vi "canDataSortSubVI.vi"(8 "canArrayID_In":string[](array[string]), 9 "canArrayDataIn":string[](array[string]), 11 "dataIn":string="         2  1FFFFFFF   00000004    8        00\t00\tFF\tFF\tFF\tFF\tFF\tFF\r\n         3  0CF101A7   00000004    8        68\t00\t97\tCC\t00\t15\t39\t1A\r\n         2  1FFFFFFF   00000004    8        00\t00\tFF\tFF\tFF\tFF\tFF\tFF\r\n         3  0CF102A7   00000004    8        30\t75\tE0\t2E\t80\tFF\tFF\tFD\r\n         3  0CF101A7   00000004    8        68\t00\t97\tCC\t00\t15\t39\t1A\r\n         2  1FFFFFFF   00000004    8        00\t00\tFF\tFF\tFF\tFF\tFF\tFF\r\n        12  1FFFFFFF   00000004    8        00\t20\tFF\tFF\tFF\tFF\tFF\tFF\r\n         3  0CF102A7   00000004    8        30\t75\tE0\t2E\t80\tFF\tFF\tFD\r\n         3  0CF101A7   00000004    8        68\t00\t97\tCC\t00\t15\t39\t1A\r\n         2  1FFFFFFF   00000004    8        00\t00\tFF\tFF\tFF\tFF\tFF\tFF\r\n        22  1FFFFFFF   00000004    8        00\t20\tFF\tFF\tFF\tFF\tFF\tFF\r\n        12  1FFFFFFF   00000004    8        00\t20\tFF\tFF\tFF\tFF\tFF\tFF\r\n         3  0CF102A7   00000004    8        30\t75\tE0\t2E\t80\tFF\tFF\tFD\r\n         3  0CF101A7   00000004    8        68\t00\t97\tCC\t00\t15\t39\t1A\r\n         2  1FFFFFFF   00000004    8        00\t00\tFF\tFF\tFF\tFF\tFF\tFF\r\n        23  0CF101A7   00000004    8        68\t00\t97\tCC\t00\t15\t39\t1B\r\n        22  1FFFFFFF   00000004    8        00\t20\tFF\tFF\tFF\tFF\tFF\tFF\r\n        12  1FFFFFFF   00000004    8        00\t20\tFF\tFF\tFF\tFF\tFF\tFF\r\n         3  0CF102A7   00000004    8        30\t75\tE0\t2E\t80\tFF\tFF\tFD\r\n         3  0CF101A7   00000004    8        68\t00\t97\tCC\t00\t15\t39\t1A\r\n         2  1FFFFFFF   00000004    8        00\t00\tFF\tFF\tFF\tFF\tFF\tFF\r\n        23  0CF102A7   00000004    8        30\t75\tE0\t2E\t80\tFF\tFF\tFD\r\n        23  0CF101A7   00000004    8        68\t00\t97\tCC\t00\t15\t39\t1B\r\n        22  1FFFFFFF   00000004    8        00\t20\tFF\tFF\tFF\tFF\tFF\tFF\r\n        12  1FFFFFFF   00000004    8        00\t20\tFF\tFF\tFF\tFF\tFF\tFF\r\n         3  0CF102A7   00000004    8        30\t75\tE0\t2E\t80\tFF\tFF\tFD\r\n         3  0CF101A7   00000004    8        68\t00\t97\tCC\t00\t15\t39\t1A\r\n         2  1FFFFFFF   00000004    8        00\t00\tFF\tFF\tFF\tFF\tFF\tFF\r\n        32  1FFFFFFF   00000004    8        00\t20\tFF\tFF\tFF\tFF\tFF\tFF\r\n        23  0CF102A7   00000004    8        30\t75\tE0\t2E\t80\tFF\tFF\tFD\r\n        23  0CF101A7   00000004    8        68\t00\t97\tCC\t00\t15\t39\t1B\r\n        22  1FFFFFFF   00000004    8        00\t20\tFF\tFF\tFF\tFF\tFF\tFF\r\n        12  1FFFFFFF   00000004    8        00\t20\tFF\tFF\tFF\tFF\tFF\tFF\r\n         3  0CF102A7   00000004    8        30\t75\tE0\t2E\t80\tFF\tFF\tFD\r\n         3  0CF101A7   00000004    8        68\t00\t97\tCC\t00\t15\t39\t1A\r\n         2  1FFFFFFF   00000004    8        00\t00\tFF\tFF\tFF\tFF\tFF\tFF\r\n        41  18F11FF0   00000004    8        FF\t3F\t90\t68\t88\t1B\t10\t8C\r\n        32  1FFFFFFF   00000004    8        00\t20\tFF\tFF\tFF\tFF\tFF\tFF\r\n        23  0CF102A7   00000004    8        30\t75\tE0\t2E\t80\tFF\tFF\tFD\r\n        23  0CF101A7   00000004    8        68\t00\t97\tCC\t00\t15\t39\t1B\r\n        22  1FFFFFFF   00000004    8        00\t20\tFF\tFF\tFF\tFF\tFF\tFF\r\n        12  1FFFFFFF   00000004    8        00\t20\tFF\tFF\tFF\tFF\tFF\tFF\r\n         3  0CF102A7   00000004    8        30\t75\tE0\t2E\t80\tFF\tFF\tFD\r\n         3  0CF101A7   00000004    8        68\t00\t97\tCC\t00\t15\t39\t1A\r\n         2  1FFFFFFF   00000004    8        00\t00\tFF\tFF\tFF\tFF\tFF\tFF\r\n        42  18F120F0   00000004    8        2B\t75\t60\tB1\tB0\t01\tFF\tFF\r\n        41  18F11FF0   00000004    8        FF\t3F\t90\t68\t88\t1B\t10\t8C\r\n        32  1FFFFFFF   00000004    8        00\t20\tFF\tFF\tFF\tFF\tFF\tFF\r\n        23  0CF102A7   00000004    8        30\t75\tE0\t2E\t80\tFF\tFF\tFD\r\n        23  0CF101A7   00000004    8        68\t00\t97\tCC\t00\t15\t39\t1B\r\n        22  1FFFFFFF   00000004    8        00\t20\tFF\tFF\tFF\tFF\tFF\tFF\r\n        12  1FFFFFFF   00000004    8        00\t20\tFF\tFF\tFF\tFF\tFF\tFF\r\n         3  0CF102A7   00000004    8        30\t75\tE0\t2E\t80\tFF\tFF\tFD\r\n         3  0CF101A7   00000004    8        68\t00\t97\tCC\t00\t15\t39\t1A\r\n         2  1FFFFFFF   00000004    8        00\t00\tFF\tFF\tFF\tFF\tFF\tFF\r\n        43  0CF101A7   00000004    8        68\t00\t97\tCC\t00\t15\t39\t1C\r\n        42  18F120F0   00000004    8        2B\t75\t60\tB1\tB0\t01\tFF\tFF\r\n        41  18F11FF0   00000004    8        FF\t3F\t90\t68\t88\t1B\t10\t8C\r\n        32  1FFFFFFF   00000004    8        00\t20\tFF\tFF\tFF\tFF\tFF\tFF") -> (1 "canArrayID":string[](array[string]), 3 "canArrayData":string[](array[string]))   [LabVIEW 2023]
panel:
  out "substring":string
  out "arrayIndex":i32
  out "whileIndex":i32
  out "index of element":i32
  out "ID":string[](array[string])
  out "Array 3":string[](array[string])
  # "VCU1:ID=0x0CF101A7"
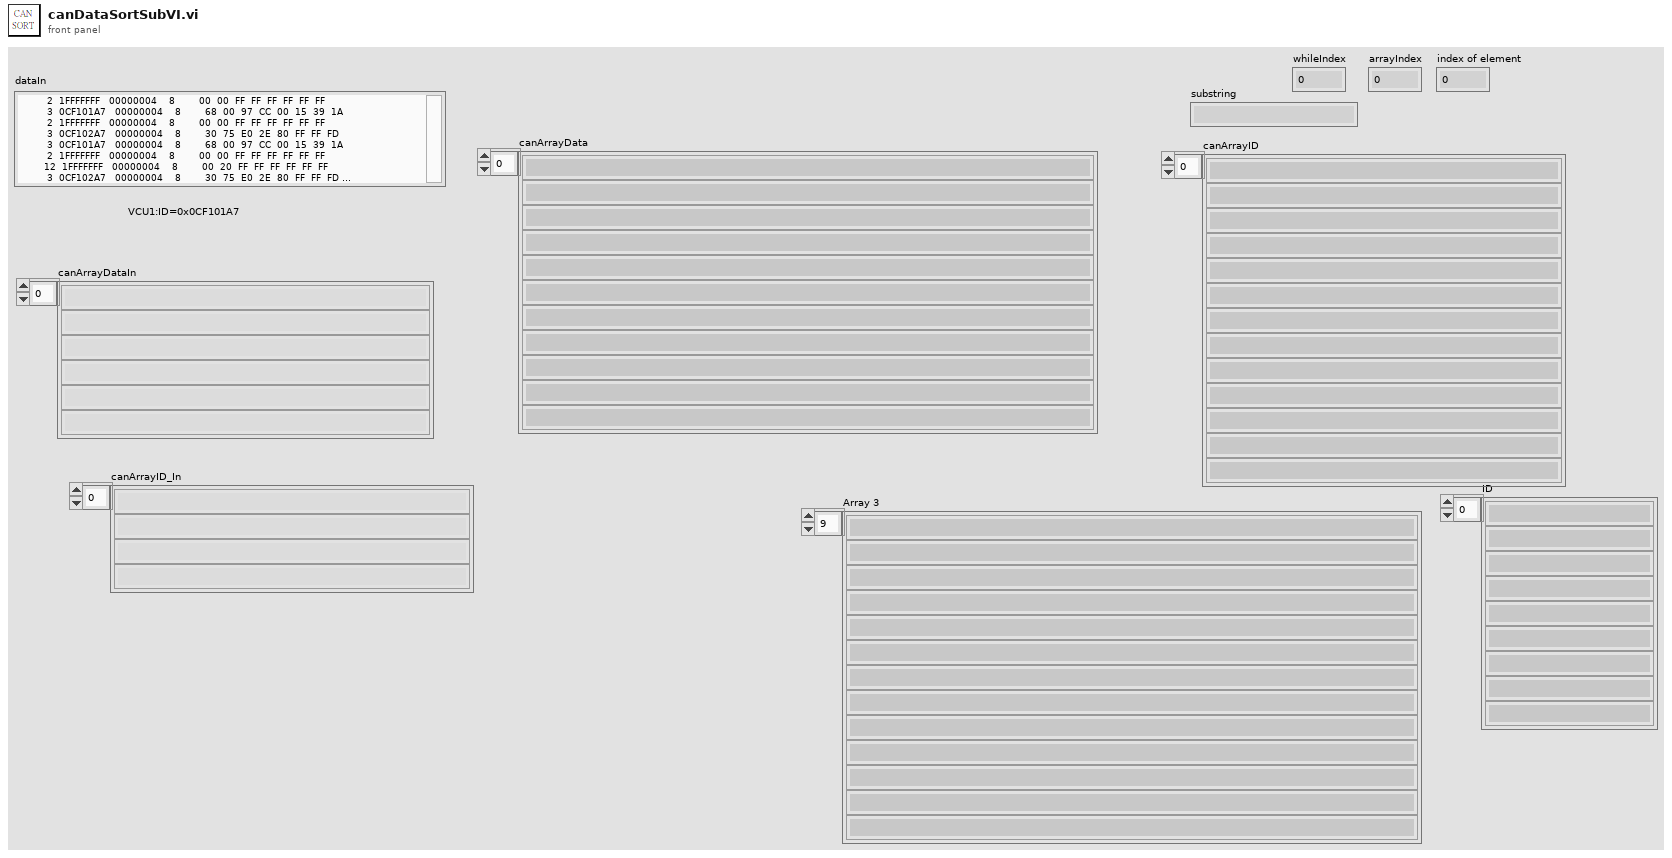
[diagram p1: front panel]
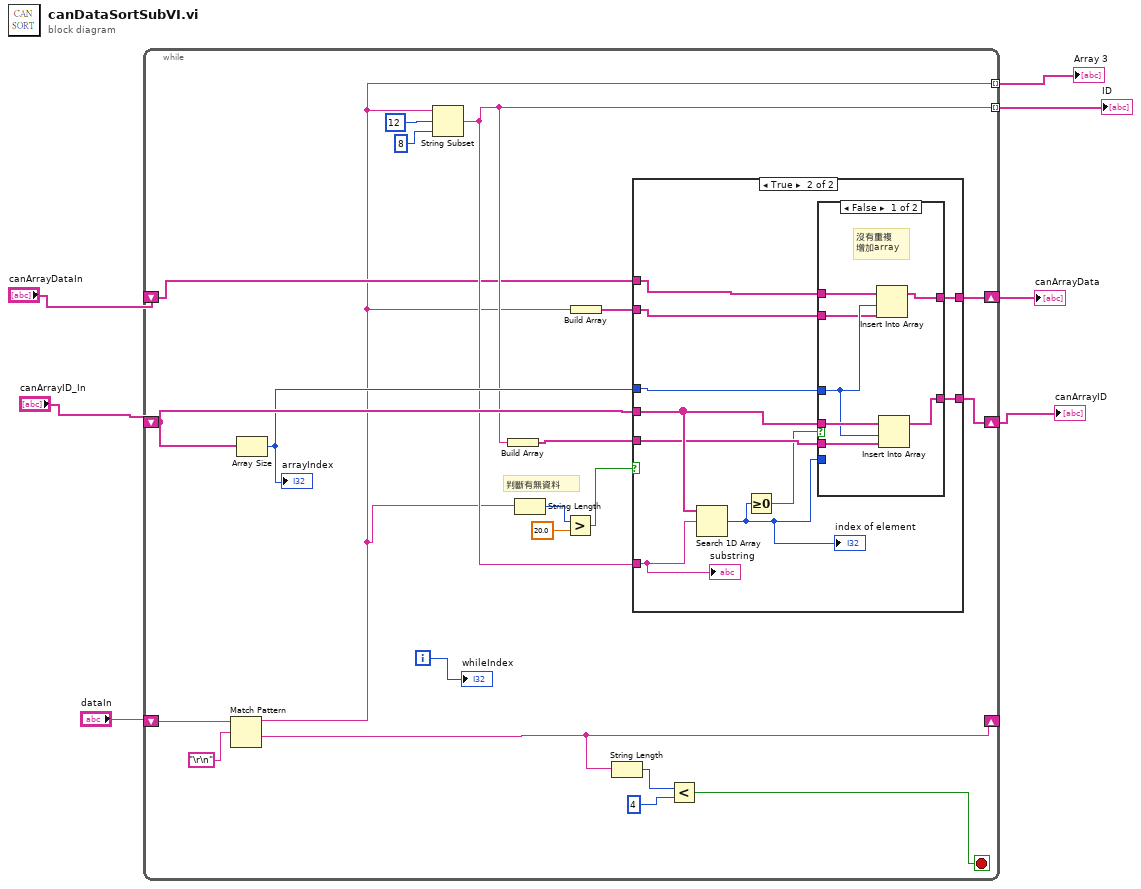
[diagram p0: block diagram]
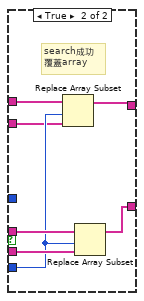
[diagram p3: hidden frame]
diagram:
  n1 = while {
    shift-right: [w27] -> _
    shift-left: "dataIn" -> [w23]
    tunnel: [w8] -> w5 mode=indexing
    tunnel: [w15] -> w4 mode=indexing
    shift-right: [w18] -> w3
    shift-left: "canArrayID_In" -> [w19]
    shift-right: [w13] -> w2
    shift-left: "canArrayDataIn" -> [w14]
    i -> [w17]
    stop <- w24 stop-if-true
    # "判斷有無資料"
    n2 = Match Pattern(string=w23, regular expression="\r\n") -> (before substring=w8:string, after substring=w27:string)  [unwired: 1 in, 2 out]
    n3 = Array Size(array=w19) -> (size(s)=w16:i32)
    "arrayIndex" <- w16
    n4 = String Subset(string=w8, offset (0)=12, length (rest)=8 ("offset (0)")) -> (substring=w15:string)
    n5 = Build Array(w15) -> (w20:string[])
    n6 = String Length(string=w8) -> (length=w11:i32)
    n7 = Greater?(x=w11, y=20.0) -> (0:w9:bool)
    n8 = Build Array(w8) -> (w12:string[])
    n9 = String Length(string=w27) -> (length=w26:i32)
    n10 = case shown="True" w9 {
      tunnel: w20 -> [_ w38]
      tunnel: w19 -> [w29 w39]
      tunnel: [w29 w40] -> w18
      tunnel: w16 -> [_ w34]
      tunnel: w15 -> [_ w37]
      tunnel: w14 -> [w30 w31]
      tunnel: [w30 w33] -> w13
      tunnel: w12 -> [_ w32]
      frame False {
      }
      frame True {
        n11 = Search 1D Array(1D array=w39, element=w37) -> (index of element=w35:i32)  [unwired: 1 in]
        "index of element" <- w35
        n12 = Greater Or Equal To 0?(x=w35) -> (x >= 0?=w36:bool)
        n13 = case shown="False" w36 {
          tunnel: [w47 w52] -> w40
          tunnel: w39 -> [w46 w54]
          tunnel: w38 -> [w45 w53]
          tunnel: w35 -> [_ w49]
          tunnel: w34 -> [w43 _]
          tunnel: [w44 w51] -> w33
          tunnel: w32 -> [w42 w48]
          tunnel: w31 -> [w41 w50]
          frame False {
            # "沒有重複\n增加array"
            n14 = Insert Into Array(array=w41, index=w43, new element=w42) -> (w44:string[])
            n15 = Insert Into Array(array=w46, index=w43, new element=w45) -> (w47:string[])
          }
          frame True {
            # "search成功\n覆蓋array"
            n16 = Replace Array Subset(array=w50, new element=w48, index=w49) -> (w51:string[])
            n17 = Replace Array Subset(array=w54, new element=w53, index=w49) -> (w52:string[])
          }
        }
        "substring" <- w37
      }
    }
    n18 = Less?(x=w26, y=4) -> (x < y?=w24:bool)
    "whileIndex" <- w17
  }
  "Array 3" <- w5
  "ID" <- w4
  "canArrayID" <- w3
  "canArrayData" <- w2
